vi "Get Panel Data.vi"(8 "error in (no error)":errorcluster, 11 "Console in":refnum<class "Console.lvclass">) -> (0 "error out":errorcluster, 2 "Panel":refnum<class "Panel Controller Interface.lvclass">, 3 "Console out":refnum<class "Console.lvclass">)   [LabVIEW 2015, in "EditPanel API.lvlib" / "Console.lvclass"]
uses:
  Console.lvclass
  Panel Control_Interface/Panel_interface/Panel Controller Interface.lvclass
  Console.lvclass/Console.ctl
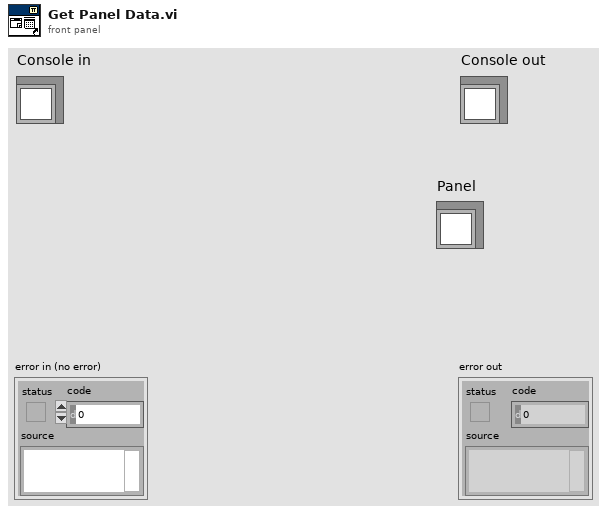
[diagram p1: front panel]
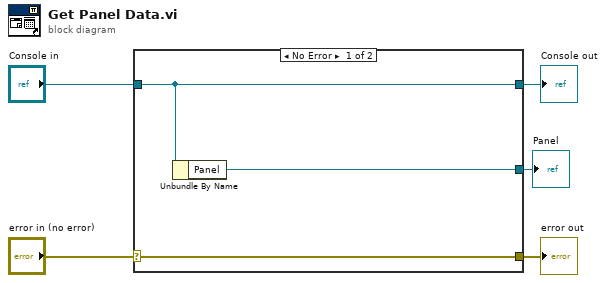
[diagram p0: block diagram]
diagram:
  n1 = case shown="No Error" "error in (no error)" {
    selector: "error in (no error)" -> [w8 w9]
    tunnel: [w8 w9] -> w4
    tunnel: [w7 w10] -> w2
    tunnel: "Console in" -> [w7 w10]
    tunnel: [w6 _] -> w1
    frame No Error {
      n2 = Unbundle By Name(w7) -> ("Panel"=w6:refnum<class "Panel Controller Interface.lvclass">)
    }
    frame Error {
    }
  }
  "error out" <- w4
  "Console out" <- w2
  "Panel" <- w1
